vi "Agilent SNA Set Trace.vi"(7 "Agilent SNA & SWP":T2, 8 "error in (no error)":errorcluster, 9 "Trace":i8=1 min=1 max=99 step=1, 10 "Channel":i8=1 min=1 max=99 step=1, 11 "VISA Resource Names":T1) -> (0 "error out":errorcluster, 3 "dup VISA Resource Names":T1)   [LabVIEW 2011]
uses:
  TypeDefs/Agilent SNA Instrument Info.ctl
  TypeDefs/Agilent SNA VISA.ctl
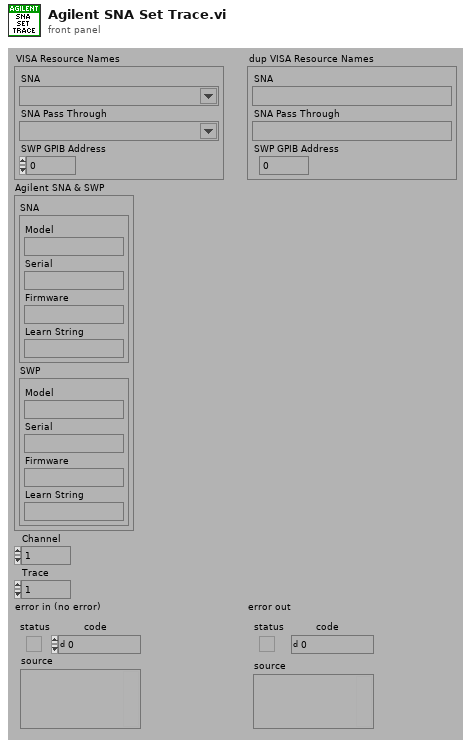
[diagram p1: front panel]
types:
  T1 = typedef "Agilent SNA VISA.ctl" = cluster{"SNA":refnum<visa-resource-name>, "SNA Pass Through":refnum<visa-resource-name>, "SWP GPIB Address":i32}
  T2 = typedef "Agilent SNA Instrument Info.ctl" = cluster{"SNA":cluster{"Model":string, "Serial":string, "Firmware":string, "Learn String":string}, "SWP":cluster{"Model":string, "Serial":string, "Firmware":string, "Learn String":string}}
  T3 = typedef "Agilent SNA Model.ctl" = enum16{"Not Supported", "8757X"}
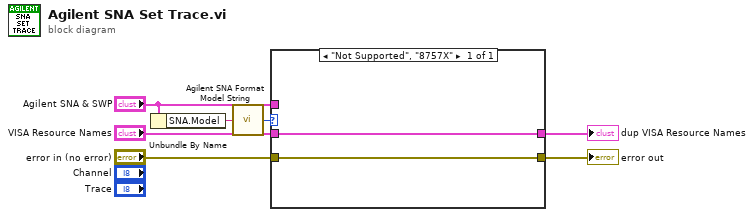
[diagram p0: block diagram]
diagram:
  n1 = Unbundle By Name("Agilent SNA & SWP") -> ("SNA.Model"=w3:string)
  n2 = call "Agilent SNA Format Model String.vi"("Model String"=w3) -> ("Model"=w1:T3)
  n3 = case shown="\"Not Supported\", \"8757X\"" w1 {
    tunnel: [w9] -> w7
    tunnel: [w8] -> w6
    tunnel: "VISA Resource Names" -> [w9]
    tunnel: "error in (no error)" -> [w8]
    tunnel: "Agilent SNA & SWP" -> [_]
    frame "Not Supported", "8757X" {
    }
  }
  "dup VISA Resource Names" <- w7
  "error out" <- w6
